vi "Sequence.SetVersion.vi"(8 "error in (no error)":errorcluster, 10 "BuildVersion":u32, 11 "RT Seq Ref":refnum<k24>) -> (0 "error out":errorcluster, 3 "RT Seq Ref out":refnum<k24>)   [LabVIEW 2015, in "Single Station Execution.lvlib"]
uses:
  Single Station Execution.lvlib
  NationalInstruments.VeriStand.RealTimeSequenceDefinitionApi
  NationalInstruments.VeriStand
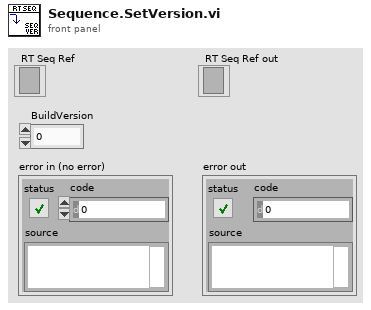
[diagram p1: front panel]
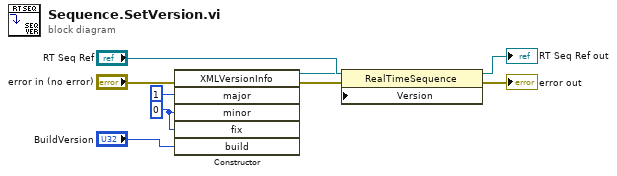
[diagram p0: block diagram]
diagram:
  w2 = u32 0 ("Fix")
  n1 = constructor class="XMLVersionInfo"(error in="error in (no error)", "major"=u32 1 ("Fix"), "minor"=w2, "fix"=w2, "build"="BuildVersion") -> (reference out=w6:refnum<k24>, error out=w7:errorcluster)  [unwired: 2 in, 5 out]
  n2 = property class="RealTimeSequence"(reference="RT Seq Ref", error in=w7, "Version"=w6) -> (reference out=→"RT Seq Ref out":refnum<k24>, error out=→"error out":errorcluster)
